vi "LV to ITX  Retrieve_SE mode  calculate R.vi"(0 "File or Folder Path":path=path "\\\\WINDYSEA\\Data/SA02835E.20160621/5_IV - sweep Bx, By, Vsg", 5 "offset":i32, 7 "length":i32=1, 9 "index":T2={"A"=3, "B"=7, "C"=5, "D"=7, "E"=3, "N1"=22, "N2"=2, "N3"=3, "N4"=4, "A 1"=8, "A 2"=10, "C 1"=5, "C 2"=1, "E 2"=4}, 11 "stop":bool=TRUE, 12 "file contains 2D data?":bool) -> (1 "Spherical coordinates":dbl[][](array[numeric])=[[2.0174217623053736, 82.16547213108355, 89.99966253494713]], 2 "long":cluster{i32[], dbl[]}(graph), 3 "G vs T":cluster{dbl[], dbl[]}(graph), 4 "A vs B":cluster{dbl[], dbl[]}[](graph), 6 "C vs D":cluster{dbl[], dbl[]}[](graph), 8 "E( = A)":dbl[][](graph)=[[0.0017692299715341491], [0.0017692136283833037], [0.0017690863023588782], [0.0017688496209154335], [0.0017685038770425205], [0.0017680499202054037], [0.0017674893850930617], [0.0017668243924686268], [0.001766058422934415], [0.0017651964716344061], [0.0017642427472359813], [0.0017632009877090636], [0.0017620750104708248], [0.0017608652742391396], [0.0017595728624556451], [0.0017582043448130663], [0.0017567662661601793], [0.0017552615750081734], [0.0017536926052565062], [0.0017520615877900346], [0.001750369446292266], [0.0017486190505704984], [0.0017468163761688894], [0.0017449663946362093], [0.0017430711585270694], [0.0017411322392178064], [0.00173915110076724], [0.0017371284502721309], [0.001735067695403663], [0.0017329740975398902], [0.0017308501525633395], [0.001728697813061485], [0.0017265191847586746], [0.0017243130979383195], [0.001722079675228934], [0.0017198237493014962], [0.0017175494357662582], [0.001715257602891662], [0.0017129477576639646], [0.0017106196150571023], [0.0017082737305671263], [0.0017059109755115484], [0.0017035339076949861], [0.0017011460381913526], [0.0016987481192410412], [0.001696340534830353], [0.0016939232673035117], [0.0016914944792014279], [0.0016890563722980509], [0.0016866135077933284], [0.0016841659562088812], [0.0016817123480454494], [0.0016792519255637455], [0.00167678239531989], [0.0016743048395971194], [0.0016718231575642846], [0.0016693380179823819], [0.0016668483136692085], [0.0016643527007184364], [0.001661849595998805], [0.0016593379257297668], [0.0016568168161481037], [0.0016542876871267801], [0.0016517529541165389], [0.001649211473357444], [0.001646662172019042], [0.0016441043883155602], [0.0016415346344120865], [0.0016389525941183341], [0.0016363616164138247], [0.0016337616268896097], [0.0016311517509948958], [0.0016285322115016994], [0.0016258992229272106], [0.0016232511517298128], [0.0016205911327671566], [0.0016179192644590148], [0.0016152343165059656], [0.0016125360700765274], [0.0016098235320753604], [0.0016070944768456592], [0.0016043474279909434], [0.0016015846317118925], [0.0015988084016285108], [0.0015960168261260111], [0.001593206925371192], [0.0015903771969006358], [0.0015875256446644787], [0.0015846519199048986], [0.0015817591421247023], [0.0015788473591891422], [0.0015759135556034417], [0.0015729565161129626], [0.0015699734610472391], [0.001566963133479985], [0.001563927240026263], [0.001560864302606199], [0.001557772515132584], [0.0015546518100495064], [0.0015515011129585568], [0.0015483186509087058], [0.0015451025280664111], [0.0015418519061765965], [0.0015385664610112705], [0.001535241571115452], [0.0015318717061404482], [0.0015284553559377148], [0.0015249878130826225], [0.0015214615773581843], [0.001517873288640703], [0.0015142172640861425], [0.001510483247947034], [0.0015066606543529205], [0.0015027371607097646], [0.0014987007425860126], [0.0014945387592606037], [0.0014902364913982847], [0.0014857805699648177], [0.0014811598431637898], [0.0014763625885140345], [0.0014713756628676013], [0.0014661880077457407], [0.0014607893102182657], [0.001455172528753526], [0.0014493349937005073], [0.0014432714402170096], [0.0014369768283609998], [0.001430450045946842], [0.001423688932632464], [0.0014166911692906376], [0.0014094582264600323], [0.0014019930241586285], [0.0013942992648841913], [0.0013863820818642153], [0.0013782439980000605], [0.001369885102234636], [0.0013613085288860498], [0.0013525184244195627], [0.0013435202698648186], [0.0013343215383315706], [0.0013249270807912919], [0.0013153429887890976], [0.0013055779770840457], [0.0012956398136702478], [0.001285534290550381], [0.0012752653997704256], [0.0012648373954012775], [0.0012542568380072875], [0.001243530490176531], [0.0012326638712340503], [0.0012216654173176143], [0.0012105435559319278], [0.0011993034971497743], [0.0011879523848188228], [0.0011764987045104994], [0.0011649468170379066], [0.0011533008341842144], [0.0011415690275172108], [0.00112975972880089], [0.0011178797231751177], [0.0011059338719710818], [0.0010939241819210522], [0.0010818517639927955], [0.0010697199980694294], [0.0010575360807087845], [0.0010453074202186766], [0.0010330374163250796], [0.0010207298994159494], [0.0010083893390998209], [0.000996015763097073], [0.000983611805239804], [0.0009711851688634172], [0.0009587401134040418], [0.0009462774820452112], [0.0009337987480185045], [0.0009213039719678584], [0.0009087955523936664], [0.0008962792641038569], [0.0008837578779581542], [0.0008712319417356349], [0.0008587018912852409], [0.0008461697809990987], [0.0008336375217772943], [0.0008211042659021054], [0.0008085699925266372], [0.0007960385032786008], [0.0007835136079844096], [0.0007709952845632046], [0.000758481525632292], [0.0007459709231387264], [0.0007334658084938012], [0.0007209718357548068], [0.0007084893537308137], [0.0006960146317669685], [0.0006835493742361976], [0.0006710940190506309], [0.000658646573323931], [0.0006462089042867589], [0.0006337826712867982], [0.000621369161660419], [0.000608969100440994], [0.0005965815300153424], [0.0005842057653796097], [0.0005718409728395344], [0.0005594858531483829], [0.0005471411540403143], [0.0005348085914800252], [0.0005224871203149015], [0.0005101749962656542], [0.0004978706486860893], [0.0004855734654269774], [0.00047328604237902835], [0.00046100770183057444], [0.0004487346500383303], [0.00043646800221623747], [0.0004242070300323999], [0.00041194798450563757], [0.00039969222094122126], [0.0003874429620111097], [0.00037520249455591677], [0.0003629730082421437], [0.00035075305472395885], [0.00033853965466073096], [0.0003263331073165443], [0.0003141309934312769], [0.00030193184870836907], [0.0002897391056501096], [0.00027755221603696786], [0.00026536928090155733], [0.00025318847133190607], [0.00024100877126632177], [0.00022883550274974585], [0.00021667051520617956], [0.00020450866112309678], [0.00019234806843691993], [0.00018018728975008414], [0.0001680249383978414], [0.00015586575472695334], [0.00014371136718485303], [0.0001315586004796784], [0.0001194094551073964], [0.00010726480050159128], [9.512232156119373e-05], [8.298375520585772e-05], [7.084909580732461e-05], [5.871731957670802e-05], [4.6588928690250314e-05], [3.4462178430546864e-05], [2.233511636835665e-05], [1.0205673639818577e-05], [-1.925858768310044e-06], [-1.4055760295897329e-05], [-2.618366395442987e-05], [-3.83126893501291e-05], [-5.044248833729508e-05], [-6.257075929598158e-05], [-7.469808617416952e-05], [-8.682601968760026e-05], [-9.895591006561838e-05], [-0.0001110889624421879], [-0.00012322366028814433], [-0.00013535807237258424], [-0.00014749303080690963], [-0.00015962808745271083], [-0.00017176295341228947], [-0.00018389892090282212], [-0.00019603543197316351], [-0.00020817127523688422], [-0.00022030680585919565], [-0.0002324433038650703], [-0.00024458105036465473], [-0.0002567185157374618], [-0.0002688538670809442], [-0.0002809898791697112], [-0.00029312908294560204], [-0.00030527155226879935], [-0.00031741978000752465], [-0.00032957225390034826], [-0.0003417248300408455], [-0.0003538773237471224], [-0.00036603268880380254], [-0.00037819450634873626], [-0.0003903630686648753], [-0.0004025336689735547], [-0.00041470267033126047], [-0.00042687155947566935], [-0.0004390398638020173], [-0.0004512061398209199], [-0.00046337405788456765], [-0.00047554627766127985], [-0.00048772183592866086], [-0.0004998996230422939], [-0.0005120786282805576], [-0.0005242600904394537], [-0.0005364427265241073], [-0.0005486240115093437], [-0.0005608064301987196], [-0.0005729902401034908], [-0.0005851734253004653], [-0.0005973563219992578], [-0.0006095390339291949], [-0.0006217207281426748], [-0.0006339033507580542], [-0.0006460867140798623], [-0.0006582657834521927], [-0.0006704395877568458], [-0.0006826098810801245], [-0.0006947780693507509], [-0.0007069475263173922], [-0.0007191199074905233], [-0.0007312931903472505], [-0.0007434654504083547], [-0.0007556365130489711], [-0.000767806831559664], [-0.0007799766471856439], [-0.0007921469039594965], [-0.000804319080109976], [-0.0008164936892732873], [-0.0008286679984362853], [-0.0008408386179972948], [-0.0008530067136029789], [-0.0008651740283836688], [-0.0008773404434133348], [-0.0008895061172716108], [-0.0009016727565713716], [-0.0009138420183186774], [-0.0009260141323432552], [-0.0009381881610898989], [-0.000950359547909883], [-0.0009625231575717245], [-0.0009746739364514011], [-0.0009868048189693535], [-0.0009989113719087645], [-0.0010109902063786713], [-0.0010230322359484388], [-0.001035025455796991], [-0.0010469583860484167], [-0.0010588176107757866], [-0.0010705885911319617], [-0.0010822576163583711], [-0.0010938116940196981], [-0.0011052369490383422], [-0.0011165192760966183], [-0.0011276457581605717], [-0.001138604311552884], [-0.0011493841682343904], [-0.0011599767148482375], [-0.0011703735801125606], [-0.0011805646954202306], [-0.0011905417588747224], [-0.001200299788909338], [-0.0012098335408801991], [-0.0012191386221804368], [-0.0012282147411115372], [-0.0012370600850891088], [-0.0012456711050970006], [-0.0012540467930224689], [-0.0012621863310856693], [-0.0012700907715429684], [-0.0012777637511643951], [-0.0012852089254229645], [-0.0012924288126067436], [-0.0012994240459889646], [-0.0013061960365705887], [-0.0013127490022867222], [-0.0013190871081203038], [-0.0013252158503701832], [-0.0013311431134570035], [-0.0013368732263969656], [-0.0013424092563833162], [-0.001347758428274114], [-0.0013529263216354257], [-0.0013579161020880178], [-0.0013627360285403082], [-0.001367393455627534], [-0.0013718916023409068], [-0.0013762349693829453], [-0.00138042776329955], [-0.001384475803767127], [-0.0013883861292625574], [-0.001392163623161993], [-0.0013958136227749441], [-0.001399341051219317], [-0.0014027489278113316], [-0.001406042595673036], [-0.0014092286483762598], [-0.0014123114924608142], [-0.0014152962845588846], [-0.0014181872159138836], [-0.0014209861285972647], [-0.0014236978485307862], [-0.0014263264722613972], [-0.0014288740098718502], [-0.0014313479762855675], [-0.001433755716259515], [-0.0014360977845500429], [-0.0014383738835270102], [-0.001440587401274777], [-0.0014427436919045497], [-0.0014448469677387464], [-0.0014468999518789738], [-0.0014489046074594592], [-0.0014508636913097058], [-0.0014527787261724451], [-0.0014546495876291395], [-0.0014564796377507841], [-0.0014582740453818162], [-0.001460036140289098], [-0.0014617673394967032], [-0.001463467649074262], [-0.001465138726333501], [-0.0014667840039662473], [-0.0014684037214867367], [-0.001469998599684956], [-0.0014715729324339573], [-0.0014731273747560988], [-0.0014746607251209076], [-0.001476175657710901], [-0.0014776753144297343], [-0.0014791610897424195], [-0.0014806348537399604], [-0.0014820977220903143], [-0.0014835489727756577], [-0.0014849881483614872], [-0.0014864143165013472], [-0.0014878265156527438], [-0.001489227782322449], [-0.001490621762892091], [-0.0014920072763653475], [-0.0014933820500876525], [-0.0014947462938155055], [-0.001496101173052073], [-0.0014974479085003594], [-0.0014987885647223854], [-0.0015001241208853794], [-0.0015014536272652816], [-0.001502776084223536], [-0.001504091049476941], [-0.0015053993504241013], [-0.0015067013563015354], [-0.001507997409936035], [-0.0015092885666887716], [-0.001510572900490721], [-0.001511848321187279], [-0.0015131165218268913], [-0.0015143785029752862], [-0.0015156348527041372], [-0.0015168875496580367], [-0.0015181337818620947], [-0.001519369332703738], [-0.001520595188014509], [-0.0015218124964138358], [-0.001523021702521801], [-0.0015242259551512918], [-0.00152542612189102], [-0.0015266195440756091], [-0.0015278044111185602], [-0.0015289801964546343], [-0.00153014880615401], [-0.0015313120008698835], [-0.0015324698075418848], [-0.0015336236462777974], [-0.0015347730873224673], [-0.0015359154413072758], [-0.0015370508608280689], [-0.0015381800478535602], [-0.0015393033421529103], [-0.0015404227695987181], [-0.0015415365081719733], [-0.0015426400807662982], [-0.0015437345803183632], [-0.0015448221158679263], [-0.0015459016659402954], [-0.0015469758928735808], [-0.0015480478071347038], [-0.0015491153085707375], [-0.0015501759991793647], [-0.001551229035111955], [-0.001552275052956365], [-0.0015533135758395802], [-0.001554340226228796], [-0.001555348915066701], [-0.001556332204602369], [-0.00155728191986208], [-0.0015581934788776446], [-0.0015590645868506425], [-0.0015598926157586001], [-0.0015606765352701238], [-0.0015614117503776896], [-0.0015620903526855907], [-0.0015627107724824761], [-0.0015632743542248757], [-0.0015637792422503927], [-0.0015642258873384697], [-0.0015646153473814629], [-0.001564944605976784], [-0.0015652110491952312], [-0.001565413996606534]], 10 "N":cluster{"N1":dbl, "N2":dbl, "N3":dbl, "N4":dbl}={"N1"=0.275, "N2"=1.998590895326537, "N3"=1.188236459055352e-05, "N4"=3.553800592300099e-05} {"N4" format="%#_6p"; "N3" format="%#_6p"; "N2" format="%#_6p"; "N1" format="%#_6p"}, 13 "Index, Wavenames":string[][](table)=[["0", "'time.SA02835E.20160621.000000'\n"], ["1", "'temp.SA02835E.20160621.000000'\n"], ["2", "'Bx.SA02835E.20160621.000000'\n"], ["3", "'By.SA02835E.20160621.000000'\n"], ["4", "'Bz.SA02835E.20160621.000000'\n"], ["5", "'Vsource.SA02835E.20160621.000000'\n"], ["6", "'Lockin0.SA02835E.20160621.000000'\n"], ["7", "'Lockin1.SA02835E.20160621.000000'\n"], ["8", "'Lockin2.SA02835E.20160621.000000'\n"], ["9", "'Lockin3.SA02835E.20160621.000000'\n"], ["10", "'Lockin4.SA02835E.20160621.000000'\n"], ["11", "'Lockin5.SA02835E.20160621.000000'\n"], ["12", "'Lockin6.SA02835E.20160621.000000'\n"], ["13", "'Lockin7.SA02835E.20160621.000000'\n"], ["14", "'B_rate.SA02835E.20160621.000000'\n"], ["15", "'DC0.SA02835E.20160621.000000'\n"], ["16", "'DC1.SA02835E.20160621.000000'\n"], ["17", "'DC2.SA02835E.20160621.000000'\n"], ["18", "'DC3.SA02835E.20160621.000000'\n"], ["19", "'DC4.SA02835E.20160621.000000'\n"], ["20", "'DC5.SA02835E.20160621.000000'\n"], ["21", "'DC6.SA02835E.20160621.000000'\n"], ["22", "'DC7.SA02835E.20160621.000000'\n"], ["23", "'V4T.SA02835E.20160621.000000'\n"], ["24", "'I.SA02835E.20160621.000000'\n"], ["", ""]], 14 "Comments":string="IGOR\nX// Date: 6/25/2016 8:10 PM\nX// sweep in plane: from theta=0 deg to 360 deg in 10 deg steps (phi=90, xy plane) @ 0.005 T/min\nX// sweep Vsg: -30mV to 275mV, 1mV steps\nX// \nX// taking lockin data between Bfield setpoints\nX// \nX// IV:\nX// low cutoff f: 0.01\nX// decimate: 10\nX// \nX// Vbg=0.57V\nX// \nX// lockin:\nX// 0: 27\nX// 1: 1 current, 3mV AC, 675uV DC, 0.4Hz\nX// 2: 2, \nX// 3: 6,\nX// 4: 7 \nX// 5: 8 current\nX// 6; 28 \nX// appliedVsg= -0.030000\n\n\n\n\n\n\n\n\n\n\n\n\n\n\n\n\n\n\n\n\n\n\n\n\n\n\n\n\n\n\n\n\n\n\n\n\n\n\n\n\n\n\n\n\n\n\n\n\n\n\n\n\nX \nX Display/R 'time.SA02835E.20160621.000000'\nX AppendToGraph 'temp.SA02835E.20160621.000000'\nX AppendToGraph 'Bx.SA02835E.20160621.000000'\nX AppendToGraph 'By.SA02835E.20160621.000000'\nX AppendToGraph 'Bz.SA02835E.20160621.000000'\nX AppendToGraph 'Vsource.SA02835E.20160621.000000'\nX AppendToGraph 'Lockin0.SA02835E.20160621.000000'\nX AppendToGraph 'Lockin1.SA02835E.20160621.000000'\nX AppendToGraph 'Lockin2.SA02835E.20160621.000000'\nX AppendToGraph 'Lockin3.SA02835E.20160621.000000'\nX AppendToGraph 'Lockin4.SA02835E.20160621.000000'\nX AppendToGraph 'Lockin5.SA02835E.20160621.000000'\nX AppendToGraph 'Lockin6.SA02835E.20160621.000000'\nX AppendToGraph 'Lockin7.SA02835E.20160621.000000'\nX AppendToGraph 'B_rate.SA02835E.20160621.000000'\nX AppendToGraph 'DC0.SA02835E.20160621.000000'\nX AppendToGraph 'DC1.SA02835E.20160621.000000'\nX AppendToGraph 'DC2.SA02835E.20160621.000000'\nX AppendToGraph 'DC3.SA02835E.20160621.000000'\nX AppendToGraph 'DC4.SA02835E.20160621.000000'\nX AppendToGraph 'DC5.SA02835E.20160621.000000'\nX AppendToGraph 'DC6.SA02835E.20160621.000000'\nX AppendToGraph 'DC7.SA02835E.20160621.000000'\nX AppendToGraph 'V4T.SA02835E.20160621.000000'\nX AppendToGraph 'I.SA02835E.20160621.000000'\nX Label bottom \"x label\"\nX Label left \"y label\"\nX ModifyGraph rgb('time.SA02835E.20160621.000000')=(65280,0,0)\nX ModifyGraph rgb('temp.SA02835E.20160621.000000')=(65280,13824,0)\nX ModifyGraph rgb('Bx.SA02835E.20160621.000000')=(65280,27648,0)\nX ModifyGraph rgb('By.SA02835E.20160621.000000')=(65280,43008,0)\nX ModifyGraph rgb('Bz.SA02835E.20160621.000000')=(65280,56832,0)\nX ModifyGraph rgb('Vsource.SA02835E.20160621.000000')=(60416,65280,0)\nX ModifyGraph rgb('Lockin0.SA02835E.20160621.000000')=(46592,65280,0)\nX ModifyGraph rgb('Lockin1.SA02835E.20160621.000000')=(32768,65280,0)\nX ModifyGraph rgb('Lockin2.SA02835E.20160621.000000')=(17408,65280,0)\nX ModifyGraph rgb('Lockin3.SA02835E.20160621.000000')=(3584,65280,0)\nX ModifyGraph rgb('Lockin4.SA02835E.20160621.000000')=(0,65280,10240)\nX ModifyGraph rgb('Lockin5.SA02835E.20160621.000000')=(0,65280,24064)\nX ModifyGraph rgb('Lockin6.SA02835E.20160621.000000')=(0,65280,37888)\nX ModifyGraph rgb('Lockin7.SA02835E.20160621.000000')=(0,65280,53248)\nX ModifyGraph rgb('B_rate.SA02835E.20160621.000000')=(0,64000,65280)\nX ModifyGraph rgb('DC0.SA02835E.20160621.000000')=(0,50176,65280)\nX ModifyGraph rgb('DC1.SA02835E.20160621.000000')=(0,36352,65280)\nX ModifyGraph rgb('DC2.SA02835E.20160621.000000')=(0,22528,65280)\nX ModifyGraph rgb('DC3.SA02835E.20160621.000000')=(0,7168,65280)\nX ModifyGraph rgb('DC4.SA02835E.20160621.000000')=(6656,0,65280)\nX ModifyGraph rgb('DC5.SA02835E.20160621.000000')=(20480,0,65280)\nX ModifyGraph rgb('DC6.SA02835E.20160621.000000')=(34304,0,65280)\nX ModifyGraph rgb('DC7.SA02835E.20160621.000000')=(48128,0,65280)\nX ModifyGraph rgb('V4T.SA02835E.20160621.000000')=(63488,0,65280)\nX ModifyGraph rgb('I.SA02835E.20160621.000000')=(65280,0,53760)\nX Legend/C/N=text0/J \"\\\\s('time.SA02835E.20160621.000000') time\\r\\\\s('temp.SA02835E.20160621.000000') temp\\r\\\\s('Bx.SA02835E.20160621.000000') Bx\\r\\\\s('By.SA02835E.20160621.000000') By\\r\\\\s('Bz.SA02835E.20160621.000000') Bz\\r\\\\s('Vsource.SA02835E.20160621.000000') Vsource\\r\\\\s('Lockin0.SA02835E.20160621.000000') Lockin0\\r\\\\s('Lockin1.SA02835E.20160621.000000') Lockin1\\r\\\\s('Lockin2.SA02835E.20160621.000000') Lockin2\\r\\\\s('Lockin3.SA02835E.20160621.000000') Lockin3\\r\\\\s('Lockin4.SA02835E.20160621.000000') Lockin4\\r\\\\s('Lockin5.SA02835E.20160621.000000') Lockin5\\r\\\\s('Lockin6.SA02835E.20160621.000000') Lockin6\\r\\\\s('Lockin7.SA02835E.20160621.000000') Lockin7\\r\\\\s('B_rate.SA02835E.20160621.000000') B_rate\\r\\\\s('DC0.SA02835E.20160621.000000') DC0\\r\\\\s('DC1.SA02835E.20160621.000000') DC1\\r\\\\s('DC2.SA02835E.20160621.000000') DC2\\r\\\\s('DC3.SA02835E.20160621.000000') DC3\\r\\\\s('DC4.SA02835E.20160621.000000') DC4\\r\\\\s('DC5.SA02835E.20160621.000000') DC5\\r\\\\s('DC6.SA02835E.20160621.000000') DC6\\r\\\\s('DC7.SA02835E.20160621.000000') DC7\\r\\\\s('V4T.SA02835E.20160621.000000') V4T\\r\\\\s('I.SA02835E.20160621.000000') I\"\nX ModifyGraph mirror(bottom)=1\nX ModifyGraph width=216\nX ModifyGraph height={Aspect,0.6}\nX ModifyGraph Log(bottom)=0\nX ModifyGraph Log(left)=0\nX \n", 15 "E index vs Field":cluster{i32[], dbl[]}(graph))   [LabVIEW 2016]
uses:
  <vilib>/Utility/miscctls.llb/LVOffsetAndMultiplierTypeDef.ctl
  <vilib>/Analysis/3filter.llb/Savitzky-Golay Filter (DBL).vi
  <vilib>/Analysis/2dsp.llb/Decimate (single shot, DBL).vi
  <vilib>/Analysis/NI_AALPro.lvlib
  <vilib>/Analysis/NI_AALBase.lvlib
panel:
  out "A or C vs N3":cluster{dbl[], dbl[]}[](graph)
  in  "A":bool
  in  "VRM mode":bool
  in  "Ring":u16(ring) items=["default", "DIFF"]
  in  "decimating factor":i32=1
  in  "decimate files":i32=1
  in  "side points":i32=6
  in  "fit points":dbl=10.0
  in  "dy/dx vs x":bool=TRUE
  in  "Portion of data":cluster{dbl, dbl}(slide)={0.75, 0.25} scale=0.0..1.0
  in  "length 2":i32=498
  in  "index 2":i32=72
  out "Ns":T1(array[cluster])=[{"N1"=0.275, "N2"=1.998590895326537, "N3"=1.188236459055352e-05, "N4"=3.553800592300099e-05}]
  in  "SE?":bool=TRUE
  in  "D  is time?":bool
  in  "B is time?":bool
  out "time":string[][](table)=[["6/25/2016", "8:10 PM"]]
  in  "Use Folder Index File?":bool
  in  "Generate Folder Index File?":bool
  in  "Ez name":string="Conductance (S)"
  in  "Ey name":string="BY (T)"
  in  "Ex name":string="Vsg (mV)"
  in  "C y name":string="voltage"
  in  "D x name":string="Vsg"
  in  "A y name":string="current"
  in  "B x name":string="Vsg"
  in  "recolor traces?":bool
  in  "Ex":T3={"Offset"=0.0, "Multiplier"=1.0}
  in  "Ey":T3={"Offset"=0.0, "Multiplier"=1.0}
  out "Path":path=path "\\\\WINDYSEA\\Data/SA02835E.20160621/5_IV - sweep Bx, By, Vsg/SA02835E.20160621.000000.itx"
  out "counter":i32
  in  "pattern":string="*.itx"
  # "A1-A2\nC1-C2\nE-E2"
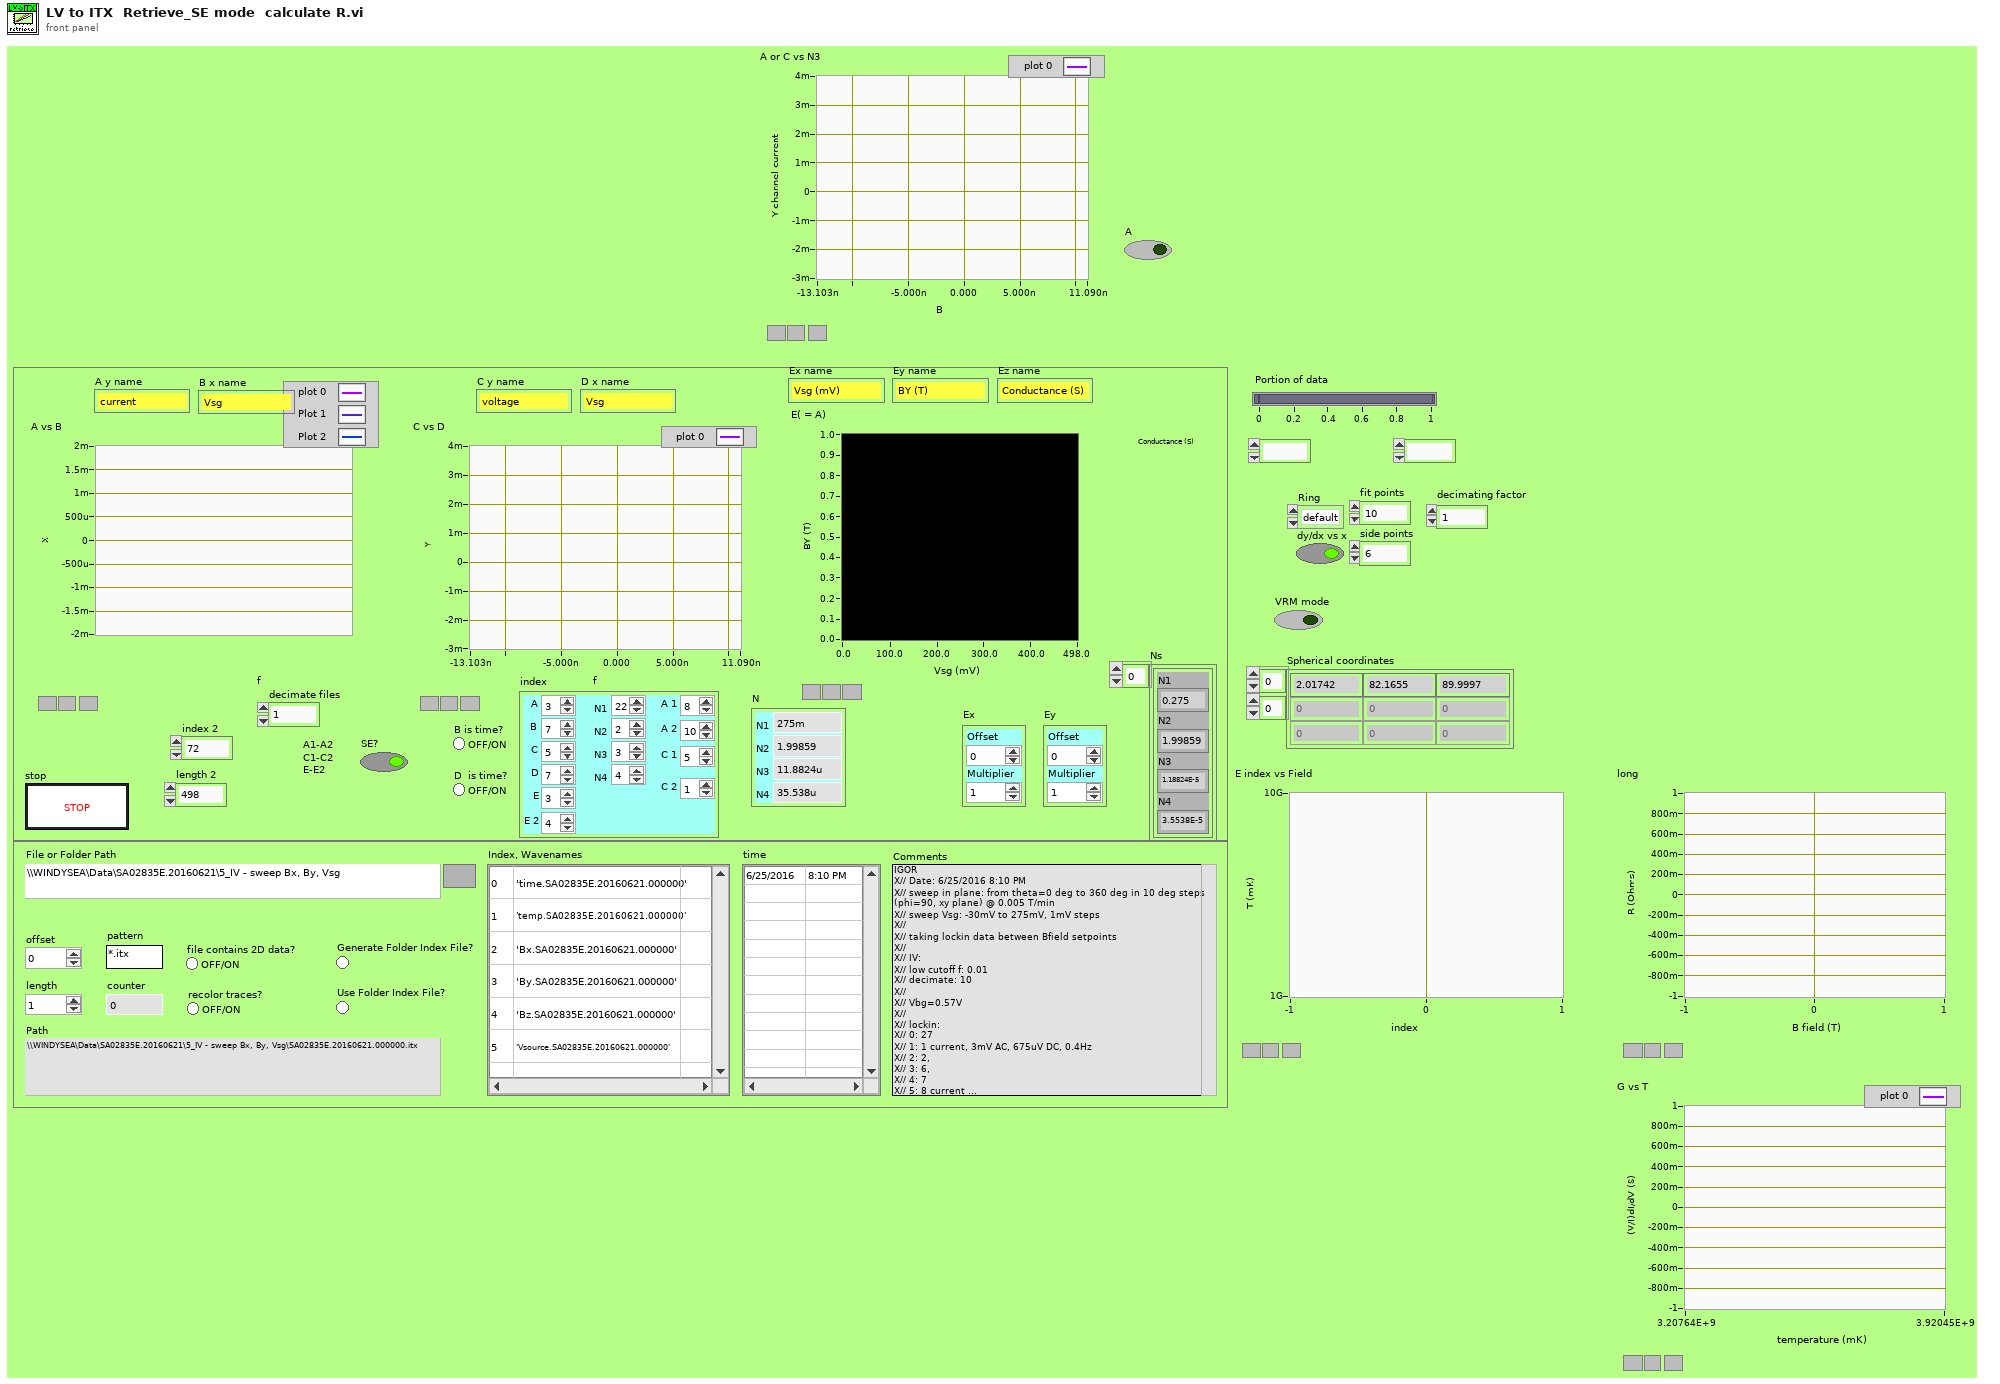
[diagram p1: front panel]
types:
  T1 = cluster{"N1":dbl, "N2":dbl, "N3":dbl, "N4":dbl}[]
  T2 = cluster{"A":i32, "B":i32, "C":i32, "D":i32, "E":i32, "N1":i32, "N2":i32, "N3":i32, "N4":i32, "A 1":i32, "A 2":i32, "C 1":i32, "C 2":i32, "E 2":i32}
  T3 = typedef "LVOffsetAndMultiplierTypeDef.ctl" = cluster{"Offset":dbl, "Multiplier":dbl}
  T4 = cluster{"Decimated Array":dbl[], "Decimated Array":dbl[]}
  T5 = cluster{"Decimated Array":dbl[], "Filtered X":dbl[]}
  T6 = cluster{"Decimated Array":dbl[], "Filtered X":dbl[]}[]
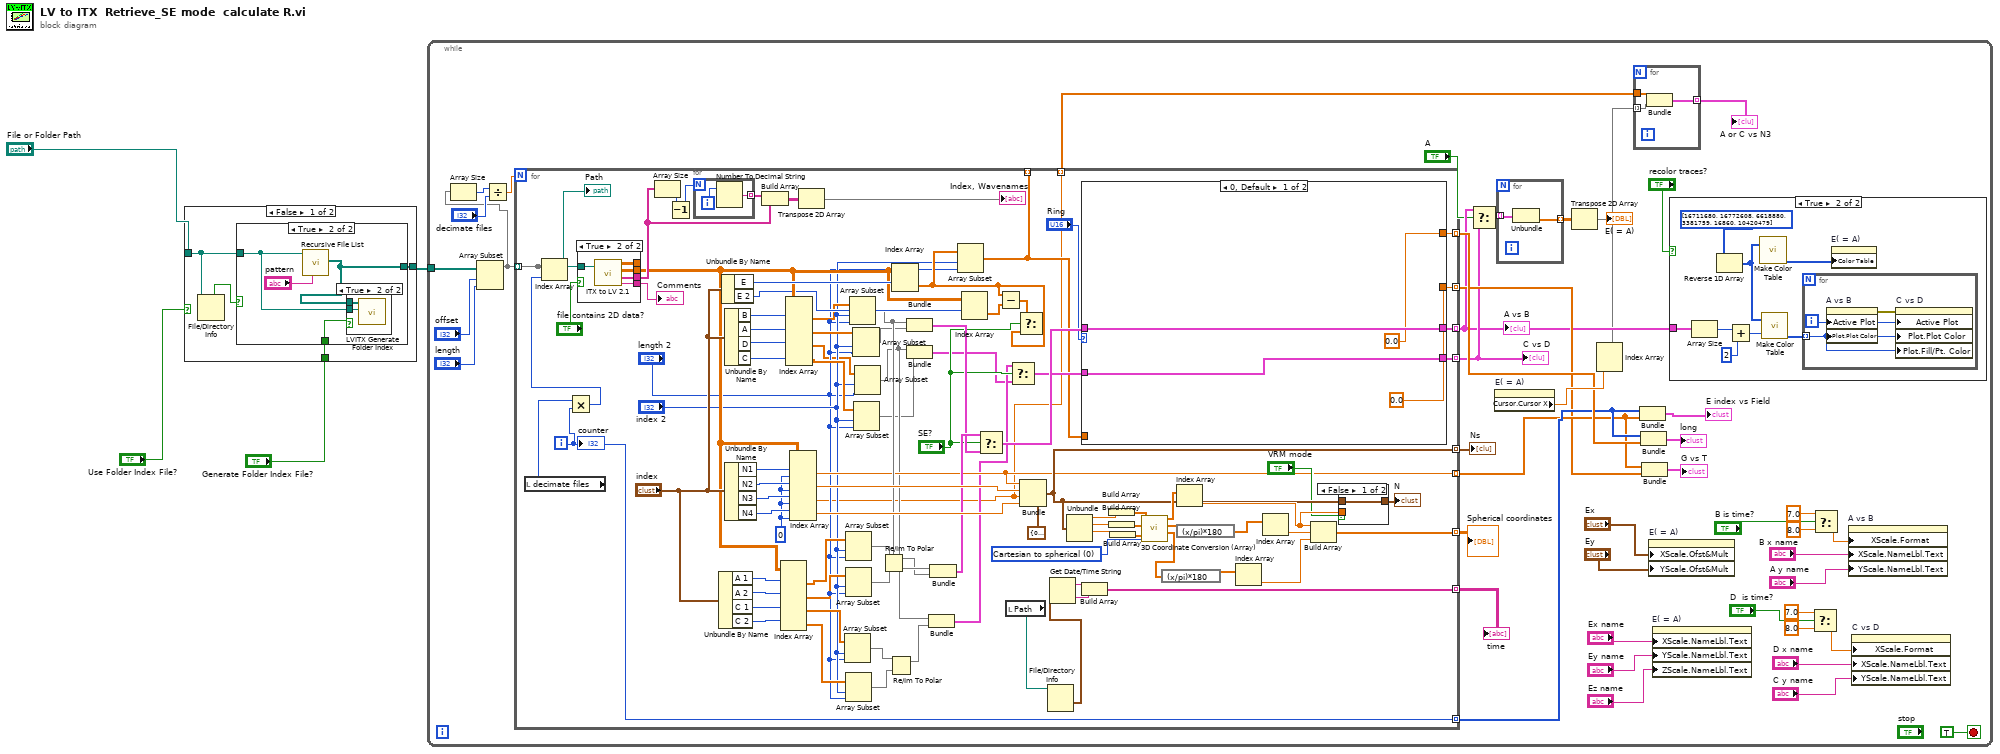
[diagram p0: block diagram]
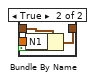
[diagram p3: hidden frame]
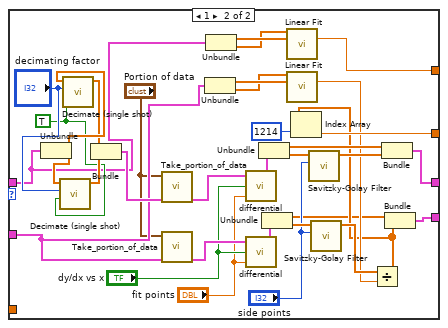
[diagram p4: hidden frame]
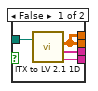
[diagram p5: hidden frame]
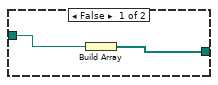
[diagram p6: hidden frame]
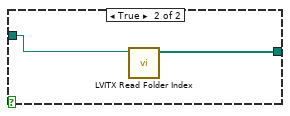
[diagram p8: hidden frame]
diagram:
  n1 = case shown="False" "Use Folder Index File?" {
    tunnel: [w6 w17] -> w2
    tunnel: "File or Folder Path" -> [w8 w18]
    tunnel: "Generate Folder Index File?" -> [w5 _]
    frame False {
      n2 = File/Directory Info(path=w8) -> (directory=w7:bool)  [unwired: 1 in, 6 out]
      n3 = case shown="True" w7 {
        tunnel: [w10 w13] -> w6
        tunnel: w8 -> [w9 w12]
        tunnel: w5 -> [_ w11]
        frame False {
          n4 = Build Array(w9) -> (w10:path[])
        }
        frame True {
          n5 = call <vilib>:"Recursive File List.vi"("pattern"="pattern", "Folder Path"=w12) -> ("All Files in Dir"=w13:path[])  [unwired: 5 in, 4 out]
          n6 = case shown="True" w11 {
            tunnel: w13 -> [_ w16]
            tunnel: w12 -> [_ w15]
            frame False {
            }
            frame True {
              n7 = call <userlib>:"LVITX Generate Folder Index.vi"("File or Folder Path"=w15, "All Files in Dir"=w16) -> ()  [unwired: 10 in]
            }
          }
        }
      }
    }
    frame True {
      n8 = call <userlib>:"LVITX Read Folder Index.vi"("File or Folder Path"=w18) -> ("Array"=w17:path[])  [unwired: 10 in]
    }
  }
  n9 = while {
    tunnel: w2 -> [w40]
    stop <- TRUE stop-if-true
    n10 = Array Subset(array=w40, index="offset", length="length") -> (w36:path[])
    n11 = Array Size(array=w36) -> (size(s)=w39:i32)
    n12 = Divide(x=w39, y="decimate files") -> (x/y=w37:dbl)
    n13 = for {
      N: w37 -> [_]
      tunnel: w36 -> [w173]
      tunnel: [w173] -> _ mode=indexing
      tunnel: [w111] -> w23 mode=indexing
      tunnel: [w110] -> w24 mode=indexing
      tunnel: [w149] -> w54 mode=indexing
      tunnel: [w100] -> w43 mode=indexing
      tunnel: [w109] -> w41 mode=indexing
      tunnel: [w103] -> w33 mode=indexing
      tunnel: [w102] -> w26 mode=indexing
      tunnel: [w97] -> w29 mode=indexing
      tunnel: [w96] -> w28 mode=indexing
      tunnel: [w81] -> _ mode=indexing
      tunnel: [w80] -> w20 mode=indexing
      i -> [w97]
      w126 = u16 0 items=["Cartesian to spherical", "spherical to Cartesian", "Cartesian to cylindrical", "cylindrical to Cartesian", "spherical to cylindrical", "cylindrical to spherical"] ("conversion type")
      w147 = 0 ("disabled index (col)")
      n14 = local read "decimate files"() -> (w106:i32)
      n15 = Multiply(x=w106, y=w97) -> (x*y=w107:i32)
      n16 = Index Array(array=w173, index=w107) -> (element=w108:path)
      "Path" <- w108
      n17 = case shown="True" "file contains 2D data?" {
        tunnel: [w222 w225] -> w174
        tunnel: [w220 w226] -> w139
        tunnel: w108 -> [w221 w227]
        tunnel: [w219 w224] -> w166
        tunnel: [w220 w223] -> _
        frame False {
          n18 = call <userlib>:"ITX to LV 2.1 1D.vi"("file (use dialog)"=w221) -> ("1D arrays"=w220:dbl[][], "wave names"=w219:string[], "Notes"=w222:string)  [unwired: 2 in]
        }
        frame True {
          n19 = call <userlib>:"ITX to LV 2.1.vi"("file (use dialog)"=w227) -> ("2D array"=w223:dbl[][], "1D arrays"=w226:dbl[][], "wave names"=w224:string[], "Notes"=w225:string)  [unwired: 1 in]
        }
      }
      "Comments" <- w174
      n20 = Array Size(array=w166) -> (size(s)=w169:i32)
      n21 = Decrement(x=w169) -> (x-1=w168:i32)
      n22 = for {
        N: w168 -> [_]
        tunnel: [w217] -> w171 mode=indexing
        i -> [w218]
        n23 = Number To Decimal String(number=w218) -> (decimal integer string=w217:string)  [unwired: 1 in]
      }
      n24 = Unbundle By Name("index") -> ("A 1"=w146:i32, "A 2"=w145:i32, "C 1"=w144:i32, "C 2"=w143:i32)
      n25 = Unbundle By Name("index") -> ("E"=w159:i32, "E 2"=w138:i32)
      n26 = Unbundle By Name("index") -> ("B"=w158:i32, "A"=w157:i32, "D"=w156:i32, "C"=w155:i32)
      n27 = Unbundle By Name("index") -> ("N1"=w160:i32, "N2"=w161:i32, "N3"=w162:i32, "N4"=w163:i32)
      n28 = Build Array(w171, w166) -> (w167:string[][])
      n29 = Index Array(array=w139, index (row) #1=w146, index (row) #2=w145, index (row) #3=w144, index (row) #4=w143) -> (element #1=w130:dbl[], element #2=w129:dbl[], element #3=w128:dbl[], element #4=w127:dbl[])  [unwired: 4 in]
      n30 = Index Array(array=w139, index (row) #1=w158, index (row) #2=w157, index (row) #3=w156, index (row) #4=w155) -> (element #1=w135:dbl[], element #2=w133:dbl[], element #3=w89:dbl[], element #4=w131:dbl[])  [unwired: 4 in]
      n31 = Index Array(array=w139, index (row) #1=w160, index (col) #1=w147, index (row) #2=w161, index (col) #2=w147, index (row) #3=w162, index (col) #3=w147, index (row) #4=w163, index (col) #4=w147) -> (element #1=w96:dbl, element #2=w153:dbl, element #3=w80:dbl, element #4=w165:dbl)
      n32 = Transpose 2D Array(2D array=w167) -> (transposed array=→"Index, Wavenames":string[][])
      n33 = Array Subset(array=w128, index="index 2", length="length 2") -> (w84:dbl[])
      n34 = Array Subset(array=w130, index="index 2", length="length 2") -> (w87:dbl[])
      n35 = Array Subset(array=w129, index="index 2", length="length 2") -> (w86:dbl[])
      n36 = Array Subset(array=w127, index="index 2", length="length 2") -> (w83:dbl[])
      n37 = Array Subset(array=w135, index="index 2", length="length 2") -> (w134:dbl[])
      n38 = Array Subset(array=w133, index="index 2", length="length 2") -> (w132:dbl[])
      n39 = Array Subset(array=w131, index="index 2", length="length 2") -> (w88:dbl[])
      n40 = Array Subset(array=w89, index="index 2", length="length 2") -> (w90:dbl[])
      n41 = Re/Im To Polar(2:w86, 3:w87) -> (1:w85:dbl[])  [unwired: 1 out]
      n42 = Re/Im To Polar(2:w83, 3:w84) -> (1:w82:dbl[])  [unwired: 1 out]
      n43 = Index Array(array=w139, index (row)=w159) -> (element=w93:dbl[])  [unwired: 1 in]
      n44 = Bundle(w134, w132) -> (w141:cluster{dbl[], dbl[]})  [unwired: 1 in]
      n45 = Bundle(w90, w88) -> (w94:cluster{dbl[], dbl[]})  [unwired: 1 in]
      n46 = Bundle(w90, w82) -> (w95:cluster{dbl[], dbl[]})  [unwired: 1 in]
      n47 = Bundle(w134, w85) -> (w142:cluster{dbl[], dbl[]})  [unwired: 1 in]
      n48 = Array Subset(array=w93, index="index 2", length="length 2") -> (w81:dbl[])
      n49 = Index Array(array=w139, index (row)=w138) -> (element=w137:dbl[])  [unwired: 1 in]
      n50 = Select(t=w142, s="SE?", f=w141) -> (s? t:f=w113:cluster{dbl[], dbl[]})
      n51 = Subtract(x=w93, y=w137) -> (x-y=w136:dbl[])
      n52 = local read "Path"() -> (w154:path)
      n53 = Select(t=w95, s="SE?", f=w94) -> (s? t:f=w112:cluster{dbl[], dbl[]})
      n54 = Select(t=w136, s="SE?", f=w93) -> ()  [unwired: 1 out]
      n55 = Bundle(cluster=cluster{"N1":dbl, "N2":dbl, "N3":dbl, "N4":dbl} {"N1"=0.0, "N2"=0.0, "N3"=0.0, "N4"=0.0}, "N1"=w96, "N2"=w153, "N3"=w80, "N4"=w165) -> (w100:cluster{"N1":dbl, "N2":dbl, "N3":dbl, "N4":dbl})
      n56 = File/Directory Info(path=w154) -> (last mod=w152:timestamp)  [unwired: 1 in, 6 out]
      n57 = Get Date/Time String(seconds (now)=w152) -> (date string=w151:string, time string=w150:string)  [unwired: 2 in]
      n58 = Unbundle(w100) -> ("N1"=w105:dbl, "N2"=w125:dbl, "N3"=w122:dbl)  [unwired: 1 out]
      n59 = case shown="0, Default" "Ring" {
        tunnel: w113 -> [w182 w200]
        tunnel: w112 -> [w181 w189]
        tunnel: [w182 w185] -> w111
        tunnel: [w181 w184] -> w110
        tunnel: [0.0 w197] -> w103
        tunnel: [0.0 w194] -> w102
        tunnel: w81 -> [_ _]
        frame 0, Default {
        }
        frame 1 {
          w201 = TRUE ("averaging")
          n60 = Unbundle(w200) -> (w206:dbl[], w204:dbl[])
          n61 = call-poly <vilib>:"Decimate (single shot).vi"("averaging"=w201, "decimating factor"="decimating factor", "X"=w204) -> ("Decimated Array"=w203:dbl[])  [unwired: 7 in, 1 out]
          n62 = call-poly <vilib>:"Decimate (single shot).vi"("averaging"=w201, "decimating factor"="decimating factor", "X"=w206) -> ("Decimated Array"=w205:dbl[])  [unwired: 7 in, 1 out]
          n63 = Bundle("Decimated Array"=w205, "Decimated Array"=w203) -> (w207:T4)  [unwired: 1 in]
          n64 = call <userlib>:"Take_portion_of_data.vi"("input IV"=w207, "Slide"="Portion of data") -> ("Output IV"=w215:cluster{dbl[], dbl[]})  [unwired: 5 in]
          n65 = call <userlib>:"Take_portion_of_data.vi"("input IV"=w189, "Slide"="Portion of data") -> ("Output IV"=w216:cluster{dbl[], dbl[]})  [unwired: 5 in]
          n66 = Unbundle(w189) -> (w198:dbl[], w193:dbl[])
          n67 = Unbundle(w200) -> (w199:dbl[], w196:dbl[])
          n68 = call <userlib>:"differential.vi"("Numeric"="fit points", "dy/dx vs x"="dy/dx vs x", "A vs B 2"=w215) -> ("A vs B 3"=w211:T4)  [unwired: 1 in]
          n69 = call <userlib>:"differential.vi"("Numeric"="fit points", "dy/dx vs x"="dy/dx vs x", "A vs B 2"=w216) -> ("A vs B 3"=w209:T4)  [unwired: 1 in]
          n70 = Unbundle(w211) -> ("Decimated Array"=w214:dbl[], "Decimated Array"=w212:dbl[])
          n71 = Unbundle(w209) -> ("Decimated Array"=w183:dbl[], "Decimated Array"=w210:dbl[])
          n72 = call <vilib>:"Linear Fit.vi"("Y"=w196, "X"=w199) -> ("slope"=w197:dbl)  [unwired: 9 in, 4 out]
          n73 = call <vilib>:"Linear Fit.vi"("Y"=w193, "X"=w198) -> ("slope"=w191:dbl)  [unwired: 9 in, 4 out]
          n74 = call-poly <vilib>:"Savitzky-Golay Filter.vi"("side points"="side points", "X"=w212) -> ("Filtered X"=w213:dbl[])  [unwired: 8 in, 1 out]
          n75 = call-poly <vilib>:"Savitzky-Golay Filter.vi"("side points"="side points", "X"=w210) -> ("Filtered X"=w192:dbl[])  [unwired: 8 in, 1 out]
          n76 = Divide(x=w192, y=w191) -> (x/y=w190:dbl[])
          n77 = Index Array(array=w190, index=1214) -> (element=w194:dbl)
          n78 = Bundle("Decimated Array"=w214, "Filtered X"=w213) -> (w185:T5)  [unwired: 1 in]
          n79 = Bundle("Decimated Array"=w183, w190) -> (w184:cluster{"Decimated Array":dbl[], dbl[]})  [unwired: 1 in]
        }
      }
      n80 = Build Array(w151, w150) -> (w149:string[])
      n81 = Build Array(w105) -> (w124:dbl[])
      n82 = Build Array(w125) -> (w123:dbl[])
      n83 = Build Array(w122) -> (w121:dbl[])
      n84 = call <vilib>:"3D Coordinate Conversion (Array).vi"("conversion type"=w126, "Axis 3"=w121, "Axis 2"=w123, "Axis 1"=w124) -> ("Axis 3 Out"=w119:dbl[], "Axis 2 Out"=w120:dbl[], "Axis 1 Out"=w118:dbl[])  [unwired: 4 in, 1 out]
      n85 = expression code="(x/pi)*180" ("degrees to radians")(w119) -> (w116:dbl[])
      n86 = Index Array(array=w118) -> (element=w101:dbl)  [unwired: 1 in]
      n87 = expression code="(x/pi)*180" ("degrees to radians")(w120) -> (w117:dbl[])
      n88 = Index Array(array=w116) -> (element=w114:dbl)  [unwired: 1 in]
      n89 = Index Array(array=w117) -> (element=w115:dbl)  [unwired: 1 in]
      n90 = Build Array(w101, w115, w114) -> (w109:dbl[])
      n91 = case shown="False" "VRM mode" {
        tunnel: w101 -> [_ w178]
        tunnel: w100 -> [w175 w177]
        tunnel: [w175 w176] -> w99
        frame False {
        }
        frame True {
          n92 = Bundle By Name(cluster=w177, "N1"=w178) -> (w176:cluster{"N1":dbl, "N2":dbl, "N3":dbl, "N4":dbl})
        }
      }
      "N" <- w99
      "counter" <- w97
    }
    "time" <- w54
    "Ns" <- w43
    "Spherical coordinates" <- w41
    "A vs B" <- w23
    "C vs D" <- w24
    n93 = Select(t=w23, s="A", f=w24) -> (s? t:f=w25:T6)
    n94 = property on="E( = A)" class="IntGraph (strict)"() -> ("Cursor.Cursor X"=w34:dbl)  [unwired: 2 in, 2 out]
    n95 = for {
      tunnel: [w68] -> w42 mode=indexing
      tunnel: [w67] -> _ mode=indexing
      tunnel: w25 -> [w67] mode=indexing
      n96 = Unbundle(w67) -> ("Filtered X"=w68:dbl[])  [unwired: 1 out]
    }
    n97 = Transpose 2D Array(2D array=w42) -> (transposed array=w21:dbl[][])
    "E( = A)" <- w21
    n98 = Index Array(array=w21, index (row)=w34) -> ()  [unwired: 1 in, 1 out]
    n99 = for {
      tunnel: w21 -> [w66] mode=indexing
      tunnel: w20 -> [w65]
      tunnel: [w64] -> w19 mode=indexing
      n100 = Bundle(w65, w66) -> (w64:cluster{dbl[], dbl[]})  [unwired: 1 in]
    }
    "A or C vs N3" <- w19
    n101 = Bundle(w29, w28) -> (→"E index vs Field":cluster{i32[], dbl[]})  [unwired: 1 in]
    n102 = Bundle(w29, w33) -> (→"long":cluster{i32[], dbl[]})  [unwired: 1 in]
    n103 = Bundle(w28, w26) -> (→"G vs T":cluster{dbl[], dbl[]})  [unwired: 1 in]
    n104 = property on="E( = A)" class="IntGraph (strict)"("XScale.Ofst&Mult"="Ex", "YScale.Ofst&Mult"="Ey") -> ()  [unwired: 2 in, 2 out]
    n105 = property on="E( = A)" class="IntGraph (strict)"("XScale.NameLbl.Text"="Ex name", "YScale.NameLbl.Text"="Ey name", "ZScale.NameLbl.Text"="Ez name") -> ()  [unwired: 2 in, 2 out]
    n106 = case shown="True" "recolor traces?" {
      tunnel: w23 -> [_ w71]
      frame False {
      }
      frame True {
        n107 = Array Size(array=w71) -> (size(s)=w72:i32)
        n108 = Reverse 1D Array(array=u32[] [16711680, 16772608, 6618880, 3381759, 16860, 10420479] ("color scale")) -> (reversed array=w70:u32[])
        n109 = Add(x=w72, y=2 ("x")) -> (x+y=w76:i32)
        n110 = call <userlib>:"Make Color Table.vi"("Array"=w70) -> ("Color Tbl"=w74:u32[])  [unwired: 1 in, 3 out]
        n111 = call <userlib>:"Make Color Table.vi"("Array"=w70, "Size/3"=w76) -> ("Color Tbl"=w73:u32[])  [unwired: 3 out]
        n112 = for {
          tunnel: w73 -> [w77] mode=indexing
          i -> [w78]
          n113 = property on="A vs B" class="XYGraph (strict)"("Active Plot"=w78, "Plot.Plot Color"=w77) -> (error out=w79:errorcluster)  [unwired: 2 in, 1 out]
          n114 = property on="C vs D" class="XYGraph (strict)"(error in=w79, "Active Plot"=w78, "Plot.Plot Color"=w77, "Plot.Fill/Pt. Color"=w77) -> ()  [unwired: 1 in, 2 out]
        }
        n115 = property on="E( = A)" class="IntGraph (strict)"("Color Table"=w74) -> ()  [unwired: 2 in, 2 out]
      }
    }
    n116 = Select(t=7.0, s="D  is time?", f=8.0) -> (s? t:f=w48:dbl)
    n117 = Select(t=7.0, s="B is time?", f=8.0) -> (s? t:f=w49:dbl)
    n118 = property on="A vs B" class="XYGraph (strict)"("XScale.Format"=w49, "XScale.NameLbl.Text"="B x name", "YScale.NameLbl.Text"="A y name") -> ()  [unwired: 2 in, 2 out]
    n119 = property on="C vs D" class="XYGraph (strict)"("XScale.Format"=w48, "XScale.NameLbl.Text"="D x name", "YScale.NameLbl.Text"="C y name") -> ()  [unwired: 2 in, 2 out]
  }
